vi "USRP Initiate and Generate (Multi).vi"(0 "niUsrpRio Sessions":T3[](array[typedef]) {"Daughterboard Clock Rate" format="%#.3pHz"; "FPGA Data Clock Rate" format="%#.3pHz"; "Data Clock Rate" format="%#.3pHz"; "Characterization Data"."Frequencies [Hz]" format="%#_6p"; "EEPROM Characterization Header"."Pointer to Device Data Header" format="%x"; "EEPROM Characterization Header"."Checksum" format="%x"; "Device Data Header"."Pointer to Characterization Data" format="%x"; "Device Data Header"."Checksum" format="%x"; "EEPROM Header"."Pointer to User Header" format="%x"; "EEPROM Header"."Pointer to Factory Header" format="%x"; "EEPROM Header"."Product Code" format="%x"; "EEPROM Header"."Checksum" format="%x"}, 1 "tx channels":T1[](array[typedef]) {"tx.coerced configurations"."coerced sample rates" format="%#.3pS/s"; "tx.coerced configurations"."coerced levels" format="%#.3gdBm"; "tx.coerced configurations"."coerced lo frequencies" format="%#.3pHz"; "tx.coerced configurations"."coerced frequencies" format="%#.3pHz"; "tx config"."channel configuration"."channel configuration"."frequency" format="%#.3pHz"; "tx config"."channel configuration"."channel configuration"."lo frequency" format="%#.3pHz"; "tx config"."channel configuration"."channel configuration"."level" format="%#_gdBm"; "tx config"."tone frequency" format="%#.3pHz"; "tx config"."sample rate" format="%#.3pS/s"}, 5 "first iteration":bool, 11 "error in":errorcluster) -> (4 "niUsrpRio Sessions (out)":T3[](array[typedef]) {"Daughterboard Clock Rate" format="%#.3pHz"; "FPGA Data Clock Rate" format="%#.3pHz"; "Data Clock Rate" format="%#.3pHz"; "Characterization Data"."Frequencies [Hz]" format="%#_6p"; "EEPROM Characterization Header"."Pointer to Device Data Header" format="%x"; "EEPROM Characterization Header"."Checksum" format="%x"; "Device Data Header"."Pointer to Characterization Data" format="%x"; "Device Data Header"."Checksum" format="%x"; "EEPROM Header"."Pointer to User Header" format="%x"; "EEPROM Header"."Pointer to Factory Header" format="%x"; "EEPROM Header"."Product Code" format="%x"; "EEPROM Header"."Checksum" format="%x"}, 15 "error out":errorcluster)   [LabVIEW 2016]
doc: "Writes baseband waveform to the device then initiates generation.\n\nVIs that must execute before this VI:\nOpen and Configure.vi\n\n<B>Input Parameters</B>\n\n<B>niUsrpRio Session</B> is the object created by the Open VI and used as the session handle for the USRP RIO design library.\n\n<B>first iteration</B> is used to determine if the device needs to be triggered. If this VI is in a loop, wire the iteration count to Equals Zero and then to this terminal. If this VI is not in a loop, wire a TRUE constant to this this terminal.\n\n<B>error in</B> describes error conditions that occur before this node runs. This input provides standard 'error in' functionality.\n\n<B>Output Parameters</B>\n\n<B>niUsrpRio Session (out)</B> is the niUsrpRio session used in all subsequent USRP RIO design library host VIs.\n\n<B>error out</B> contains error information. This output provides standard 'error out' functionality."
uses:
  <instrlib>/niUsrpRio/Config/v1/Host/Public/niUsrpRio Session.ctl
  <instrlib>/_niInstr/Register Bus/v0/Host/Public/Register Bus Session.ctl
  <instrlib>/_niInstr/Register Bus/v0/Host/Private/Session Data.ctl
  <instrlib>/niUsrpRio/Config/v1/Host/Private/DB Queue Reference.ctl
  <instrlib>/niUsrpRio/Config/v1/Host/Private/Daughterboard Data.ctl
  <instrlib>/niUsrpRio/Config/v1/Host/Private/ATR state data.ctl
  <instrlib>/niUsrpRio/Config/v1/Host/Private/Antenna Configuration.ctl
  <instrlib>/niUsrpRio/Config/v1/Host/Private/CPLD Power Mode.ctl
  <instrlib>/niUsrpRio/Config/v1/Host/Public/EEPROM Header.ctl
  <instrlib>/niUsrpRio/Config/v1/Host/Public/EEPROM Device Data Header.ctl
  <instrlib>/niUsrpRio/Config/v1/Host/Public/EEPROM Characterization Header.ctl
  <instrlib>/niUsrpRio/Config/v1/Host/Public/Characterization Data.ctl
  <instrlib>/niUsrpRio/Config/v1/Host/Public/IQ Imbalance.ctl
  USRP Tx Channels.ctl
  USRP Start Trigger.ctl
  <instrlib>/_niInstr/Register Bus/v0/Host/niInstr Register Bus v0 Host.lvlib
  <instrlib>/niUsrpRio/Config/v1/Host/niUsrpRio Config v1 Host.lvlib
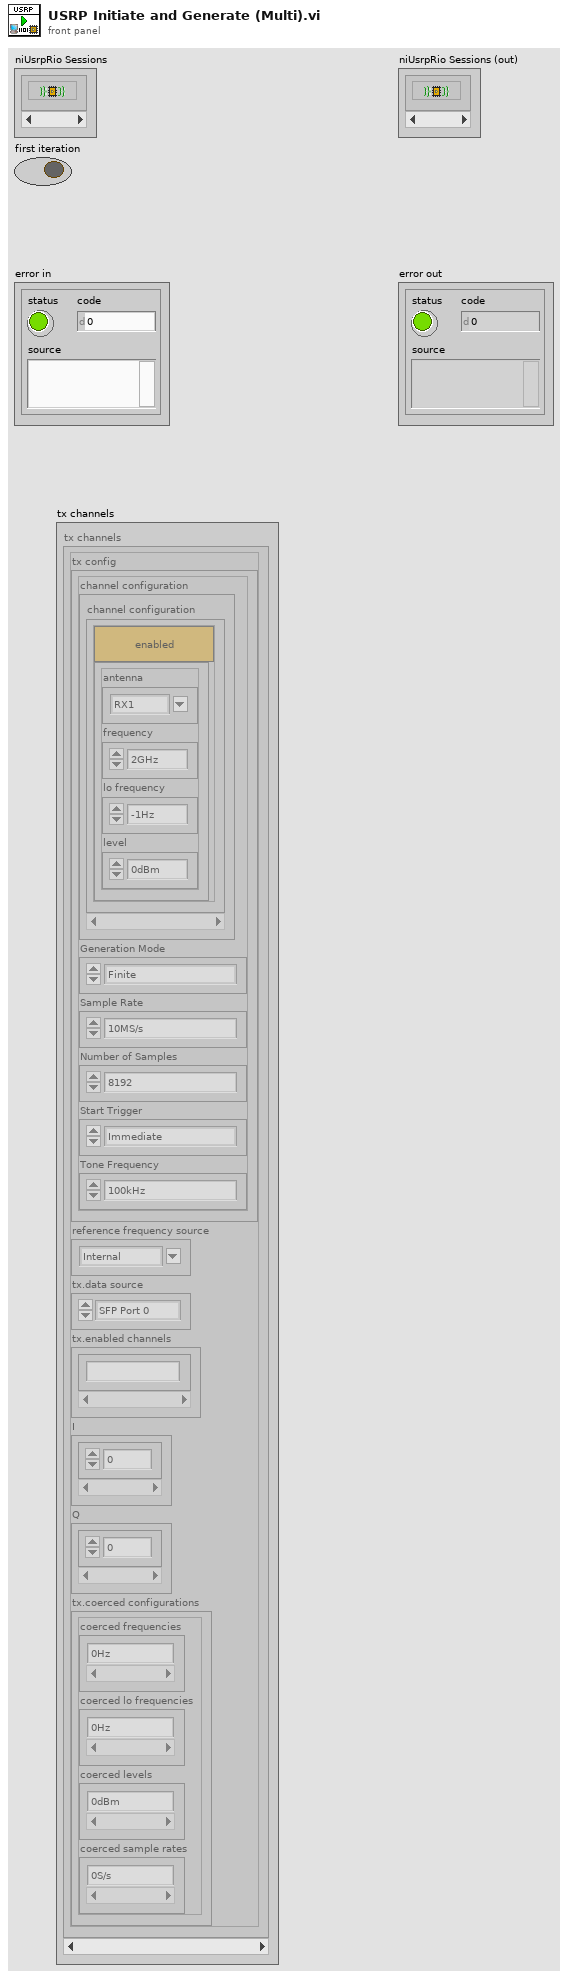
[diagram p1: front panel]
types:
  T1 = typedef "USRP Tx Channels.ctl" = cluster{"tx config":cluster{"channel configuration":cluster{"channel enable":bool, "channel configuration":cluster{"antenna":string, "frequency":dbl, "lo frequency":dbl, "level":dbl}}[], "transfer mode":enum16{"Finite", "Continuous"}, "sample rate":dbl, "number of samples":u32, "start trigger":T2, "tone frequency":dbl}, "reference frequency source":string, "tx.data source":enum16{"SFP Port 0", "SFP Port 1", "Host"}, "tx.enabled channels":string[], "I":i16[], "Q":i16[], "tx.coerced configurations":cluster{"coerced frequencies":dbl[], "coerced lo frequencies":dbl[], "coerced levels":dbl[], "coerced sample rates":dbl[]}}
  T2 = typedef "USRP Start Trigger.ctl" = enum8{"Software", "Digital Edge", "Rx Start Trigger", "Tx Start Trigger", "Immediate", "Future Time Event"}
  T3 = typedef "niUsrpRio Config v1 Host.lvlib/niUsrpRio Session.ctl" = cluster{"FPGA Interface":refnum<k20>, "RIO Interface Number":u32, "Data Clock Rate":u32, "FPGA Data Clock Rate":u32, "Global Settings Register Bus":T4, "Radio 0 Settings Register Bus":T4, "Radio 1 Settings Register Bus":T4, "Radio Settings Bus Semaphore":T5, "DB Queues":T6[], "Characterization Data Valid?":bool, "EEPROM Header":T7, "Device Data Header":T8, "EEPROM Characterization Header":T9, "Characterization Data":T10[], "FPGA Current Version":u32, "FPGA Oldest Compatible Version":u32, "Fixed Logic Current Version":u32, "Fixed Logic Oldest Compatible Version":u32, "FPGA Radio Settings Bus Current Version":u32, "FPGA Radio Settings Bus Oldest Compatible Version":u32, "FPGA Board Config Current Version":u32, "FPGA Board Config Oldest Compatible Version":u32, "Daughterboard Clock Rate":u32, "daughterboard configuration session handles":u64[]}
  T4 = typedef "niInstr Register Bus v0 Host.lvlib/Register Bus Session.ctl" = refnum<queue>
  T5 = typedef "Semaphore RefNum" = refnum<k1>
  T6 = typedef "niUsrpRio Config v1 Host.lvlib/DB Queue Reference.ctl" = refnum<queue>
  T7 = typedef "niUsrpRio Config v1 Host.lvlib/EEPROM Header.ctl" = cluster{"Checksum":u32, "Product Code":u16, "Hardware Current Version":u16, "Hardware Oldest Compatible Version":u16, "EEPROM Map Current Version":u16, "EEPROM Map Oldest Compatible Version":u16, "User Password":string, "Pointer to Factory Header":u32, "Pointer to User Header":u32, "Recommended Interval":u16, "Number of Reserved Bytes":i32, "Number of Daughterboards":u8, "Daughterboard IDs":u16[], "Daughterboard Serial Numbers":string[]}
  T8 = typedef "niUsrpRio Config v1 Host.lvlib/EEPROM Device Data Header.ctl" = cluster{"Checksum":u32, "Number of Channels":u8, "Number of Gain Settings":u16[], "Pointer to Characterization Data":u32[], "Number of Reserved Bytes":i32, "Number of Frequencies":u16[]}
  T9 = typedef "niUsrpRio Config v1 Host.lvlib/EEPROM Characterization Header.ctl" = cluster{"Checksum":u32, "Date":timestamp, "Temperature":sgl, "Misc. Info":string, "Pointer to Device Data Header":u32, "Number of Reserved Bytes":i32}
  T10 = typedef "niUsrpRio Config v1 Host.lvlib/Characterization Data.ctl" = cluster{"Gains[dB]":dbl[], "Frequencies [Hz]":dbl[], "IQ Imbalance Table":T11[], "Measured Gains[dB]":dbl[][]}
  T11 = typedef "niUsrpRio Config v1 Host.lvlib/IQ Imbalance.ctl" = cluster{"Gain Imbalance [linear]":dbl, "Phase Imbalance [radians]":dbl, "Offset":cdb}
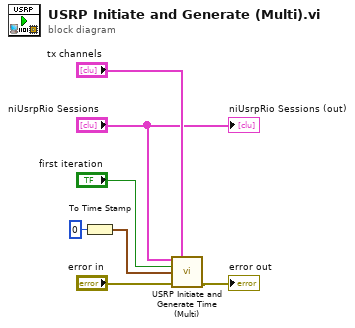
[diagram p0: block diagram]
diagram:
  n1 = To Time Stamp(1:0) -> (0:w3:timestamp)
  n2 = call "USRP Initiate and Generate Time (Multi).vi"("niUsrpRio Sessions"="niUsrpRio Sessions", "tx channels"="tx channels", "first iteration"="first iteration", "start trigger time"=w3, "error in"="error in") -> ("error out"=→"error out":errorcluster)  [unwired: 9 in, 1 out]
  "niUsrpRio Sessions (out)" <- "niUsrpRio Sessions"
